vi "0-ch1.vi"(3 "this":i32, 4 "button":i32, 5 "shift in":bool, 6 "settings in":T1={"Auto1"=TRUE, "Auto2"=TRUE, "Rel1"=TRUE, "Rel2"=TRUE, "Filt1"=TRUE, "Filt2"=TRUE, "Rate"=enum."Med", "Range1"=enum."10mV", "Range2"=enum."100mV", "Filt3"=TRUE, "Filt4"=TRUE, "Rel temp"=TRUE, "Analog1"=FALSE, "Analog2"=FALSE, "Analog temp"=FALSE, "Digital1"=TRUE, "Digital2"=TRUE, "Digital temp "=TRUE, "Window1"=enum."0,01%", "Window2"=enum."0,01%", "Window temp"=enum."0,01%", "RDGS1"="010", "RDGS2"="010", "RDGS temp"="010", "Type_type1"=TRUE, "Type_type2"=TRUE, "Type_type temp"=TRUE, "LSync"=FALSE, "Unit"=enum."C", "Sens"=TRUE, "Type tcoupl"=enum."J", "Junc"=TRUE}) -> (0 "next state":i32, 1 "shift out":bool, 2 "settings out":T1)   [LabVIEW 2017]
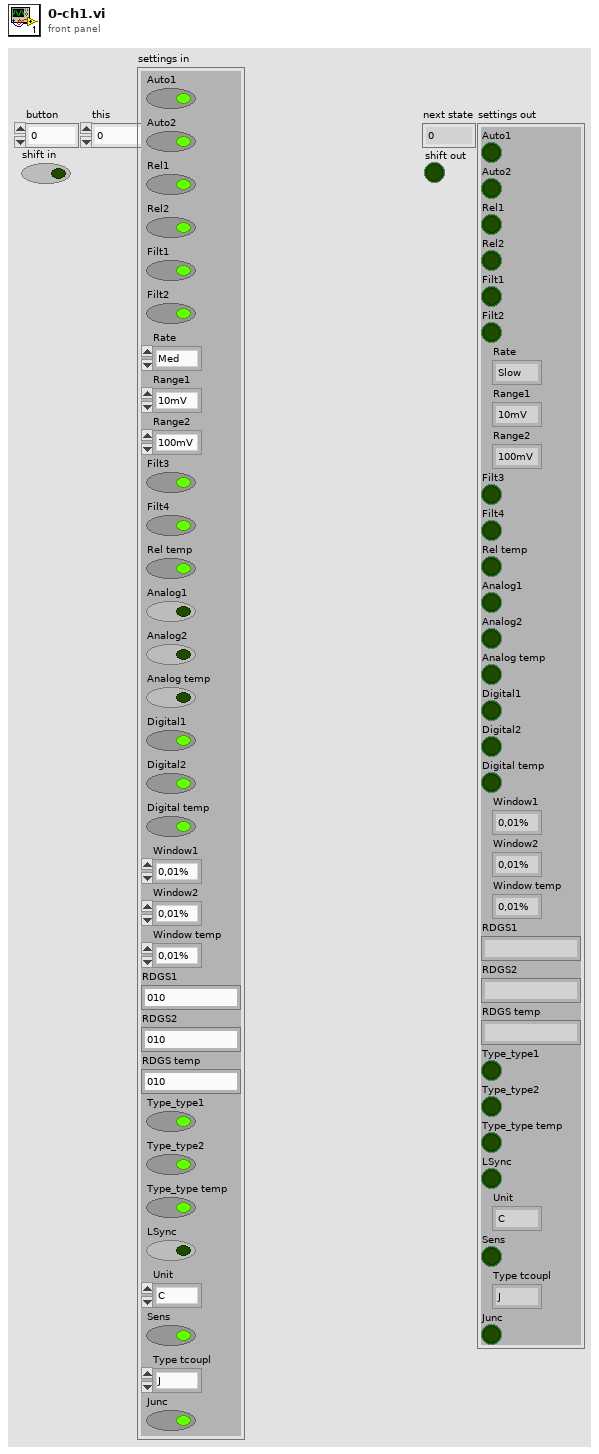
[diagram p1: front panel]
types:
  T1 = cluster{"Auto1":bool, "Auto2":bool, "Rel1":bool, "Rel2":bool, "Filt1":bool, "Filt2":bool, "Rate":enum16{"Slow", "Med", "Fast"}, "Range1":enum16{"10mV", "100mV", "1V", "10V", "100V"}, "Range2":enum16{"100mV", "1V", "10V"}, "Filt3":bool, "Filt4":bool, "Rel temp":bool, "Analog1":bool, "Analog2":bool, "Analog temp":bool, "Digital1":bool, "Digital2":bool, "Digital temp ":bool, "Window1":enum16{"0,01%", "0,1%", "1%", "10%", "None"}, "Window2":enum16{"0,01%", "0,1%", "1%", "10%", "None"}, "Window temp":enum16{"0,01%", "0,1%", "1%", "10%", "None"}, "RDGS1":string, "RDGS2":string, "RDGS temp":string, "Type_type1":bool, "Type_type2":bool, "Type_type temp":bool, "LSync":bool, "Unit":enum16{"C", "K", "F"}, "Sens":bool, "Type tcoupl":enum16{"J", "K", "T", "E", "R", "S", "B", "N"}, "Junc":bool}
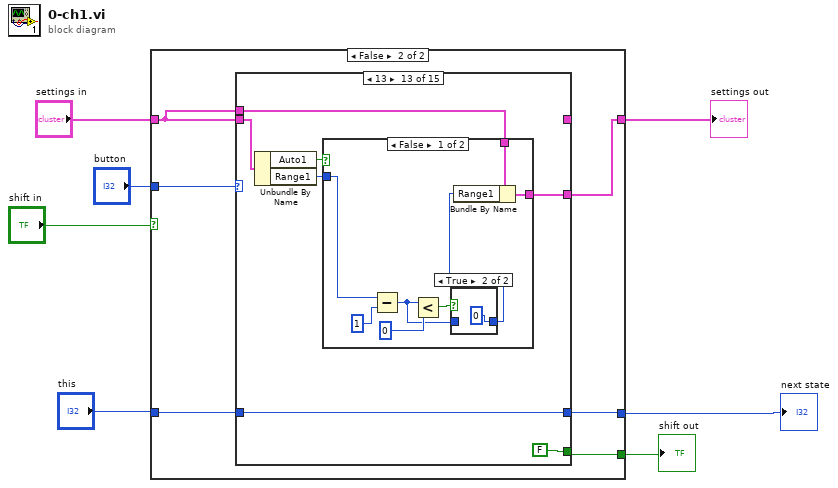
[diagram p0: block diagram]
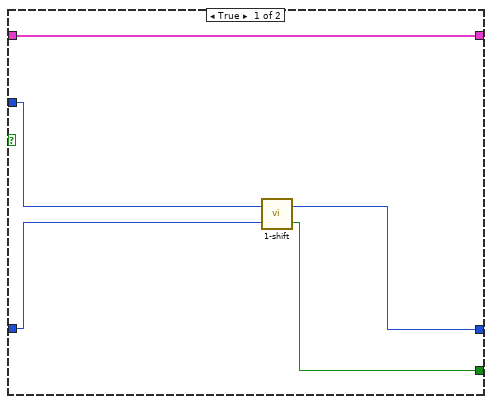
[diagram p2: hidden frame]
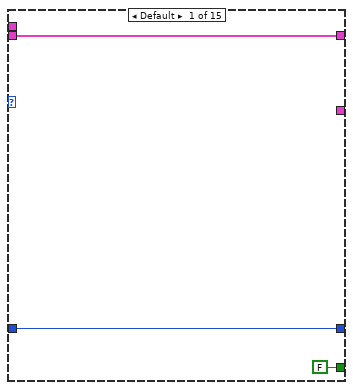
[diagram p3: hidden frame]
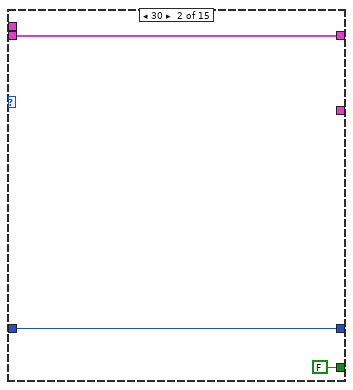
[diagram p4: hidden frame]
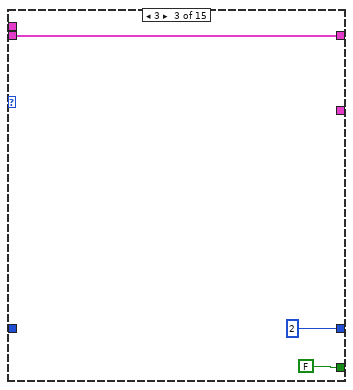
[diagram p5: hidden frame]
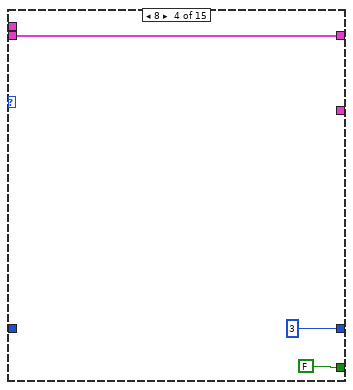
[diagram p6: hidden frame]
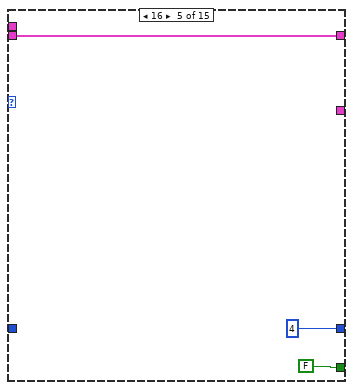
[diagram p7: hidden frame]
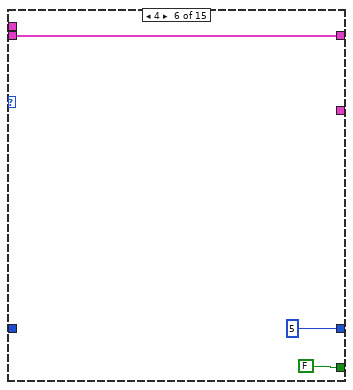
[diagram p8: hidden frame]
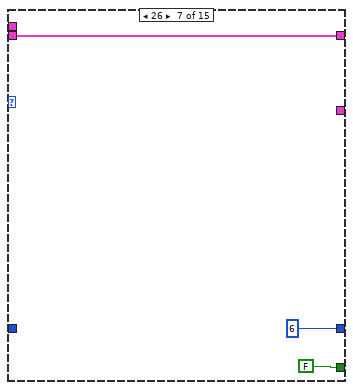
[diagram p9: hidden frame]
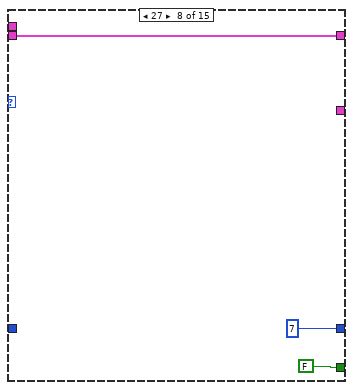
[diagram p10: hidden frame]
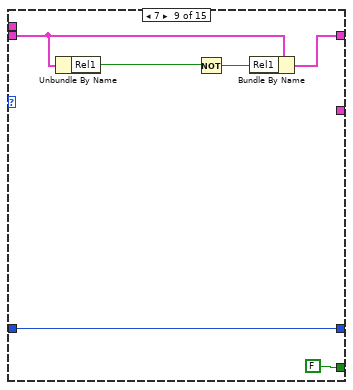
[diagram p11: hidden frame]
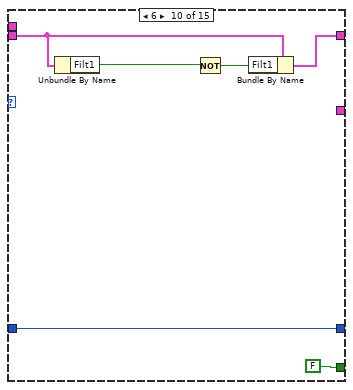
[diagram p12: hidden frame]
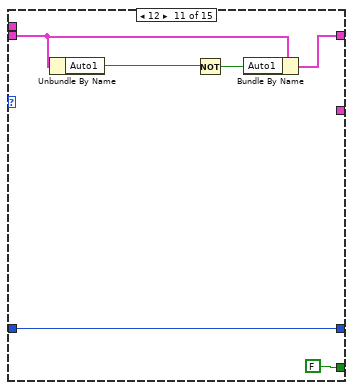
[diagram p13: hidden frame]
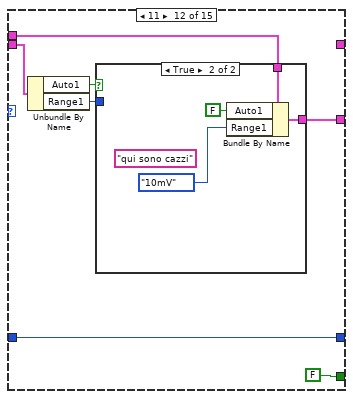
[diagram p14: hidden frame]
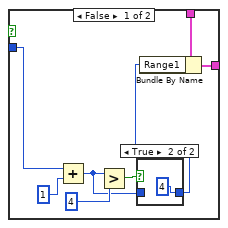
[diagram p15: hidden frame]
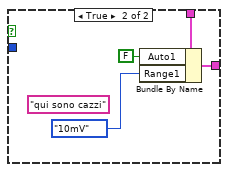
[diagram p18: hidden frame]
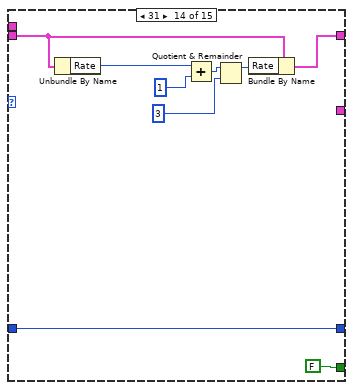
[diagram p19: hidden frame]
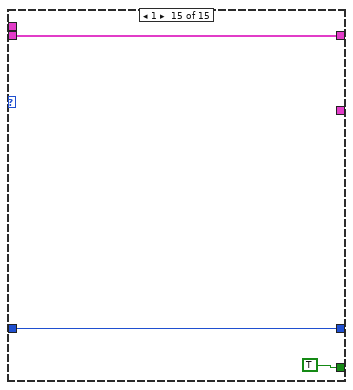
[diagram p20: hidden frame]
diagram:
  n1 = case shown="False" "shift in" {
    tunnel: "button" -> [w12 w18]
    tunnel: [w11 w17] -> w5
    tunnel: "this" -> [w10 w16]
    tunnel: [w8 w15] -> w3
    tunnel: "settings in" -> [w9 w14]
    tunnel: [w9 w13] -> w2
    frame True {
      n2 = call "1-shift.vi"("this"=w10, "button"=w12) -> ("shift"=w8:bool, "next state"=w11:i32)
    }
    frame False {
      n3 = case shown="13" w18 {
        tunnel: [w20 w23 2 3 4 5 6 7 w47 w53 w59 w66 w87 w110 w114] -> w17
        tunnel: w16 -> [w20 w23 _ _ _ _ _ _ w47 w53 w59 w66 w87 w110 w114]
        tunnel: [FALSE ("shift") FALSE ("shift") FALSE ("shift") FALSE ("shift") FALSE ("shift") FALSE ("shift") FALSE ("shift") FALSE ("shift") FALSE ("shift") FALSE ("shift") FALSE ("shift") FALSE ("shift") FALSE ("shift") FALSE ("shift") TRUE ("shift")] -> w15
        tunnel: w14 -> [w21 w24 w25 w28 w31 w34 w37 w40 w44 w50 w56 w65 w86 w109 w112]
        tunnel: [w21 w24 w25 w28 w31 w34 w37 w40 w43 w49 w55 _ _ w108 w112] -> _
        tunnel: w14 -> [_ _ _ _ _ _ _ _ _ _ _ w63 w84 _ _]
        tunnel: [_ _ _ _ _ _ _ _ _ _ _ w62 w83 _ _] -> w13
        frame Default {
        }
        frame 30 {
        }
        frame 3 {
        }
        frame 8 {
        }
        frame 16 {
        }
        frame 4 {
        }
        frame 26 {
        }
        frame 27 {
        }
        frame 7 {
          n4 = Unbundle By Name(w44) -> ("Rel1"=w46:bool)
          n5 = Not(x=w46) -> (.not. x?=w45:bool)
          n6 = Bundle By Name(cluster=w44, "Rel1"=w45) -> (w43:T1)
        }
        frame 6 {
          n7 = Unbundle By Name(w50) -> ("Filt1"=w52:bool)
          n8 = Not(x=w52) -> (.not. x?=w51:bool)
          n9 = Bundle By Name(cluster=w50, "Filt1"=w51) -> (w49:T1)
        }
        frame 12 {
          n10 = Unbundle By Name(w56) -> ("Auto1"=w58:bool)
          n11 = Not(x=w58) -> (.not. x?=w57:bool)
          n12 = Bundle By Name(cluster=w56, "Auto1"=w57) -> (w55:T1)
        }
        frame 11 {
          n13 = Unbundle By Name(w65) -> ("Auto1"=w64:bool, "Range1"=w61:enum16{"10mV", "100mV", "1V", "10V", "100V"})
          n14 = case shown="True" w64 {
            tunnel: w63 -> [w74 w81]
            tunnel: [w73 w80] -> w62
            tunnel: w61 -> [w71 _]
            frame False {
              n15 = Add(x=w71, y=1) -> (x+y=w69:i32)
              n16 = Greater?(x=w69, y=4) -> (0:w70:bool)
              n17 = case shown="True" w70 {
                tunnel: w69 -> [w76 _]
                tunnel: [w76 4] -> w68
                frame False {
                }
                frame True {
                }
              }
              n18 = Bundle By Name(cluster=w74, "Range1"=w68) -> (w73:T1)
            }
            frame True {
              (unwired) "qui sono cazzi"
              n19 = Bundle By Name(cluster=w81, "Auto1"=FALSE, "Range1"=enum16{"10mV", "100mV", "1V", "10V", "100V"}."10mV") -> (w80:T1)
            }
          }
        }
        frame 13 {
          n20 = Unbundle By Name(w86) -> ("Auto1"=w85:bool, "Range1"=w82:enum16{"10mV", "100mV", "1V", "10V", "100V"})
          n21 = case shown="False" w85 {
            tunnel: w84 -> [w95 w102]
            tunnel: [w94 w101] -> w83
            tunnel: w82 -> [w92 _]
            frame False {
              n22 = Subtract(x=w92, y=1) -> (x-y=w90:i32)
              n23 = Less?(x=w90, y=0) -> (x < y?=w91:bool)
              n24 = case shown="True" w91 {
                tunnel: w90 -> [w97 _]
                tunnel: [w97 0] -> w89
                frame False {
                }
                frame True {
                }
              }
              n25 = Bundle By Name(cluster=w95, "Range1"=w89) -> (w94:T1)
            }
            frame True {
              (unwired) "qui sono cazzi"
              n26 = Bundle By Name(cluster=w102, "Auto1"=FALSE, "Range1"=enum16{"10mV", "100mV", "1V", "10V", "100V"}."10mV") -> (w101:T1)
            }
          }
        }
        frame 31 {
          n27 = Unbundle By Name(w109) -> ("Rate"=w107:enum16{"Slow", "Med", "Fast"})
          n28 = Add(x=w107, y=1) -> (x+y=w105:i32)
          n29 = Quotient & Remainder(x=w105, y=3) -> (x-y*floor(x/y)=w104:i32)  [unwired: 1 out]
          n30 = Bundle By Name(cluster=w109, "Rate"=w104) -> (w108:T1)
        }
        frame 1 {
        }
      }
    }
  }
  "next state" <- w5
  "shift out" <- w3
  "settings out" <- w2
